vi "Read Icon.vi"(8 "error in (no error)":errorcluster, 11 "SampleDescriptionHolder in":refnum<class "MetaDataObj.lvclass">) -> (0 "error out":errorcluster, 2 "Icon":picture, 3 "SampleDescriptionHolder out":refnum<class "MetaDataObj.lvclass">)   [LabVIEW 2016, in "MetaDataObj.lvclass"]
uses:
  <resource>/dialog/NewProjectWizard/MetaDataObj/MetaDataObj.lvclass
  <resource>/dialog/NewProjectWizard/MetaDataObj/MetaDataObj.lvclass/MetaDataObj.ctl
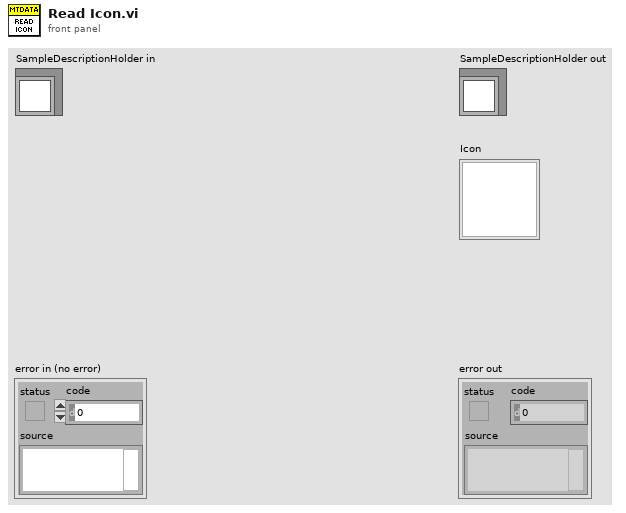
[diagram p1: front panel]
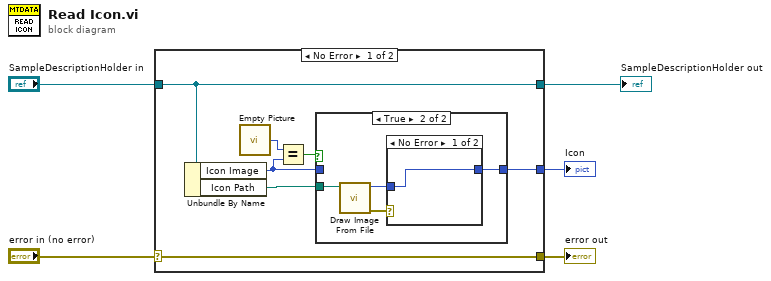
[diagram p0: block diagram]
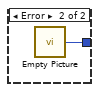
[diagram p3: hidden frame]
diagram:
  n1 = case shown="No Error" "error in (no error)" {
    selector: "error in (no error)" -> [w12 w20]
    tunnel: [w12 w20] -> w4
    tunnel: [w11 w21] -> w2
    tunnel: "SampleDescriptionHolder in" -> [w11 w21]
    tunnel: [w6 _] -> w1
    frame No Error {
      n2 = Unbundle By Name(w11) -> ("Icon Image"=w9:picture, "Icon Path"=w7:path)
      n3 = call "Empty Picture"() -> ("empty picture"=w10:picture)
      n4 = Equal?(x=w10, y=w9) -> (x = y?=w8:bool)
      n5 = case shown="True" w8 {
        tunnel: w9 -> [w13 _]
        tunnel: w7 -> [_ w17]
        tunnel: [w13 w14] -> w6
        frame False {
        }
        frame True {
          n6 = call <resource>:"Draw Image From File.vi"("Image Path In"=w17) -> ("error out"=w16:errorcluster, "Picture Out"=w15:picture)  [unwired: 9 in]
          n7 = case shown="No Error" w16 {
            tunnel: w15 -> [w18 _]
            tunnel: [w18 w19] -> w14
            frame No Error {
            }
            frame Error {
              n8 = call "Empty Picture"() -> ("empty picture"=w19:picture)
            }
          }
        }
      }
    }
    frame Error {
    }
  }
  "error out" <- w4
  "SampleDescriptionHolder out" <- w2
  "Icon" <- w1
